vi "WPI_SolenoidDoesDevRefExist.vi"(0 "SolenoidDevRefArray":T1[](array[typedef]), 7 "SolenoidDevRef":T1={"DevStatus"={"status"=FALSE, "code"=0, "source"=""}, "Pneumatics Control Module"=1, "Forward Solenoid Channel"=enum."Solenoid 1", "Reverse Solenoid Channel"=enum."Invalid"}) -> (4 "index":i32, 8 "exists":bool)   [LabVIEW 2017]
doc: "This is used to find the index of a DevRef within an array of DevRefs."
uses:
  <vilib>/Rock Robotics/WPI/Solenoid/WPI_SolenoidDevRef.ctl
  <vilib>/Rock Robotics/WPI/Solenoid/WPI_SolenoidChannel.ctl
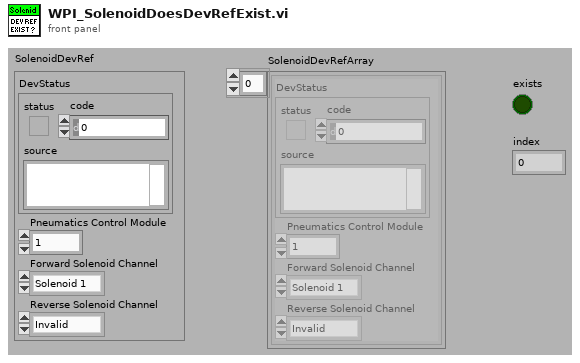
[diagram p1: front panel]
types:
  T1 = typedef "WPI_SolenoidDevRef.ctl" = cluster{"DevStatus":errorcluster, "Pneumatics Control Module":u8, "Forward Solenoid Channel":T2, "Reverse Solenoid Channel":T2}
  T2 = typedef "WPI_SolenoidChannel.ctl" = enum8{"Solenoid 0", "Solenoid 1", "Solenoid 2", "Solenoid 3", "Solenoid 4", "Solenoid 5", "Solenoid 6", "Solenoid 7", "Invalid"}
  T3 = cluster{"Pneumatics Control Module":u8, "Forward Solenoid Channel":T2}
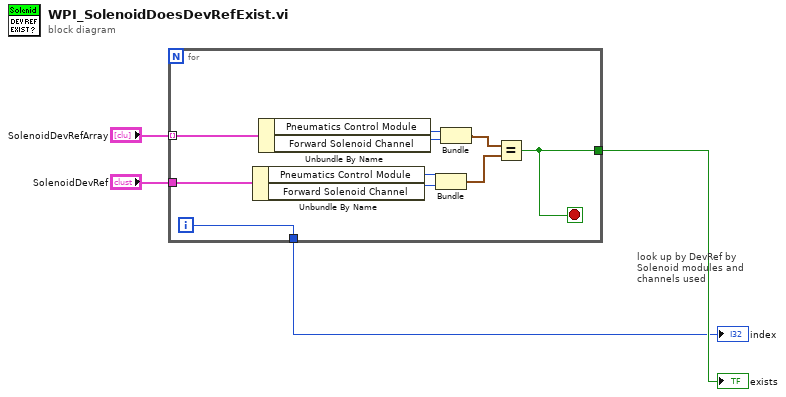
[diagram p0: block diagram]
diagram:
  # "look up by DevRef by Solenoid modules and channels used"
  n1 = for {
    tunnel: "SolenoidDevRefArray" -> [w14] mode=indexing
    tunnel: "SolenoidDevRef" -> [w13]
    tunnel: [w5] -> w2
    tunnel: [w6] -> w1
    i -> [w6]
    stop <- w5 stop-if-true
    n2 = Unbundle By Name(w13) -> ("Pneumatics Control Module"=w10:u8, "Forward Solenoid Channel"=w9:T2)
    n3 = Unbundle By Name(w14) -> ("Pneumatics Control Module"=w12:u8, "Forward Solenoid Channel"=w11:T2)
    n4 = Bundle("Pneumatics Control Module"=w10, "Forward Solenoid Channel"=w9) -> (w8:T3)  [unwired: 1 out]
    n5 = Bundle("Pneumatics Control Module"=w12, "Forward Solenoid Channel"=w11) -> (w7:T3)  [unwired: 1 out]
    n6 = Equal?(x=w7, y=w8) -> (x = y?=w5:bool)
  }
  "exists" <- w2
  "index" <- w1
